vi "libget_input_uuid.vi"(8 "error in (no error)":errorcluster, 11 "input":i32) -> (0 "error out":errorcluster, 3 "UUID":string)   [LabVIEW 2015]
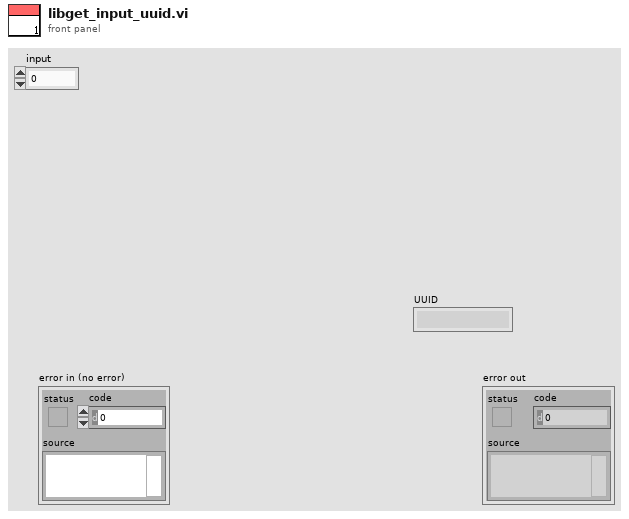
[diagram p1: front panel]
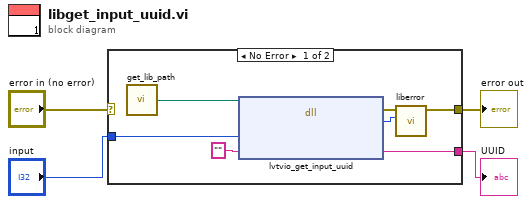
[diagram p0: block diagram]
diagram:
  n1 = case shown="No Error" "error in (no error)" {
    selector: "error in (no error)" -> [_ w12]
    tunnel: [w5 w12] -> w2
    tunnel: [w9 _] -> w4
    tunnel: "input" -> [w8 _]
    frame No Error {
      n2 = call "get_lib_path.vi"() -> ("Path"=w11:path)
      n3 = dll-call lib="S:/thingiverselv/lib/win_x64/libthingiverseio.dll" fn="lvtvio_get_input_uuid"(path in=w11, "input"=w8, "UUID"="" ("result")) -> (error out=w7:errorcluster, "return type"=w6:i32, "UUID"=w9:string)  [unwired: 3 in, 1 out]
      n4 = call "liberror.vi"("tvio errors"=w6, "error in (no error)"=w7) -> ("error out"=w5:errorcluster)  [unwired: 9 in]
    }
    frame Error {
    }
  }
  "error out" <- w2
  "UUID" <- w4
